vi "Plot-Data.vi"(8 "Reset Plot":bool, 10 "Y":dbl[](array[numeric]), 11 "X":dbl[](array[numeric])) -> (2 "Spectrum":cluster{"X":dbl[], "Y":dbl[]}[](graph))   [LabVIEW 2009]
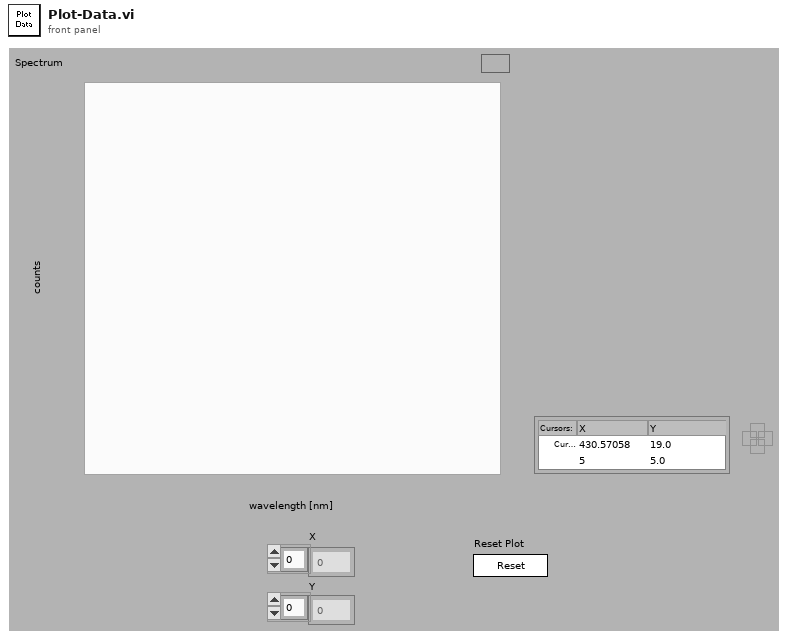
[diagram p1: front panel]
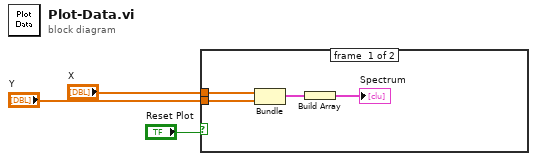
[diagram p0: block diagram]
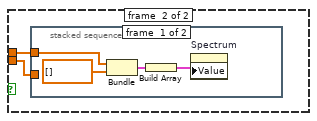
[diagram p2: hidden frame]
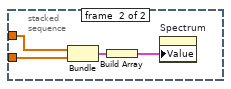
[diagram p3: hidden frame]
diagram:
  n1 = case shown="False" "Reset Plot" {
    tunnel: "X" -> [w7 w9]
    tunnel: "Y" -> [w6 w8]
    frame #0 {
      n2 = Bundle("X"=w7, "Y"=w6) -> (w5:cluster{"X":dbl[], "Y":dbl[]})  [unwired: 1 in]
      n3 = Build Array(w5) -> (→"Spectrum":cluster{"X":dbl[], "Y":dbl[]}[])
    }
    frame #1 {
      n4 = stacked-sequence {
        tunnel: w9 -> [w12 w17]
        tunnel: w8 -> [_ w16]
        frame #0 {
          n5 = Bundle("X"=w12, dbl[] []) -> (w11:cluster{"X":dbl[], dbl[]})  [unwired: 1 in]
          n6 = Build Array(w11) -> (w10:cluster{"X":dbl[], dbl[]}[])
          n7 = property on="Spectrum" class="XYGraph (strict)"("Value"=w10) -> ()  [unwired: 2 in, 2 out]
        }
        frame #1 {
          n8 = Bundle("X"=w17, "Y"=w16) -> (w15:cluster{"X":dbl[], "Y":dbl[]})  [unwired: 1 in]
          n9 = Build Array(w15) -> (w14:cluster{"X":dbl[], "Y":dbl[]}[])
          n10 = property on="Spectrum" class="XYGraph (strict)"("Value"=w14) -> ()  [unwired: 2 in, 2 out]
        }
      }
    }
  }
